vi "Twist_Create.vi"(9 "dTHETA":dbl, 10 "dY":dbl, 11 "dX":dbl) -> (3 "TWIST":T1)   [LabVIEW 2019, in "Trajectory_Library.lvlib"]
doc: "Constructs a Twist2d with the given values.\n\nA change in distance along arc since the last pose update. We can use ideas from differential calculus to create new Pose2ds from a Twist2d and vise versa.\n\nParameters:\n - dx - Change in x direction relative to robot.\n - dy - Change in y direction relative to robot.\n - dtheta - Change in angle relative to robot.\n\nResults:\n - TWIST - TWIST data structure"
uses:
  Trajectory_Library.lvlib
  TWIST2D.ctl
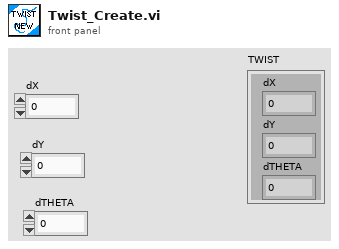
[diagram p1: front panel]
types:
  T1 = typedef "Trajectory_Library.lvlib/TWIST2D.ctl" = cluster{"dX":dbl, "dY":dbl, "dTHETA":dbl}
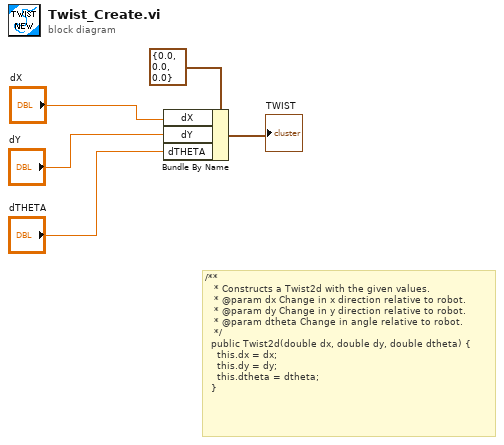
[diagram p0: block diagram]
diagram:
  # "/**\n   * Constructs a Twist2d with the given values.\n   * @param dx Change in x direction relative to robot.\n   * @param dy Change in y direction relative to robot.\n   * @param dtheta Change in angle relative to robot.\n   */\n  public Twist2d(double dx, double dy, double dtheta) {\n    this.dx = dx;\n    this.dy = dy;\n    this.dtheta = dtheta;\n  }"
  n1 = Bundle By Name(cluster=T1 {"dX"=0.0, "dY"=0.0, "dTHETA"=0.0} ("TWIST"), "dX"="dX", "dY"="dY", "dTHETA"="dTHETA") -> (→"TWIST":T1)
